vi "LOER_GetImage.vi"(0 "XRef":T5, 1 "State In":T3={"Inputs"=1, "SelectedIndex"=1, "ClassInfo"=[], "Width"=100, "EventReg Type"=variant}) -> (14 "Image":T2, 15 "Fatal Error Out":T1)   [LabVIEW 2016, in "LV Object Event Registration Node.xnode"]
uses:
  LV Object Event Registration Node.xnode
  <vilib>/XNodeSupport/XNodeXNodeRef.ctl
  LOER_State.ctl
  LOER_ClassInfo.ctl
  <vilib>/XNodeSupport/XNodeImage.ctl
  <vilib>/XNodeSupport/XNodeErrorCluster.ctl
  <vilib>/XNodeSupport/NI_XNodeSupport.lvlib
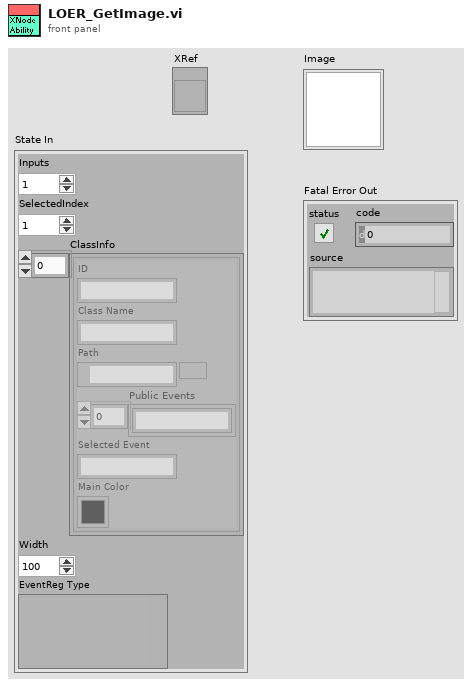
[diagram p1: front panel]
types:
  T1 = typedef "NI_XNodeSupport.lvlib/XNodeErrorCluster.ctl" = errorcluster
  T2 = typedef "NI_XNodeSupport.lvlib/XNodeImage.ctl" = picture
  T3 = typedef "LV Object Event Registration Node.xnode/LOER_State.ctl" = cluster{"Inputs":u16, "SelectedIndex":i16, "ClassInfo":T4[], "Width":u16, "EventReg Type":variant}
  T4 = typedef "LV Object Event Registration Node.xnode/LOER_ClassInfo.ctl" = cluster{"ID":string, "Class Name":string, "Path":path, "Public Events":string[], "Selected Event":string, "Main Color":u32}
  T5 = typedef "NI_XNodeSupport.lvlib/XNodeXNodeRef.ctl" = refnum<vi>
  T6 = cluster{"horizontal":enum16{"left", "center", "right"}, "vertical":enum16{"top", "center", "bottom"}}
  T7 = cluster{"left":i16, "top":i16, "right":i16, "bottom":i16}
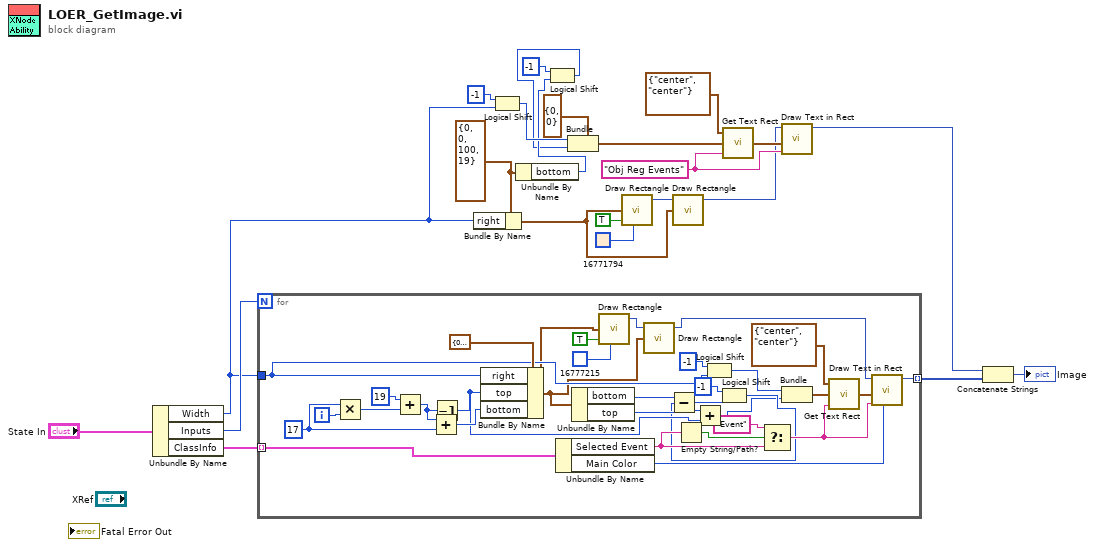
[diagram p0: block diagram]
diagram:
  w12 = "Obj Reg Events" ("text")
  w4 = T7 {"left"=0, "top"=0, "right"=100, "bottom"=19} ("rect")
  n1 = Unbundle By Name("State In") -> ("Width"=w8:u16, "Inputs"=w22:u16, "ClassInfo"=w17:T4[])
  n2 = for {
    N: w22 -> [_]
    tunnel: [w51] -> w18 mode=indexing
    tunnel: w17 -> [w41] mode=indexing
    tunnel: w8 -> [w33]
    i -> [w50]
    w45 = 17 ("x")
    n3 = Multiply(x=w45, y=w50) -> (x*y=w49:i32)
    n4 = Add(x=19, y=w49) -> (x+y=w46:i32)
    n5 = Add(x=w46, y=w45) -> (x+y=w44:i32)
    n6 = Decrement(x=w46) -> (x-1=w27:i32)
    n7 = Bundle By Name(cluster=T7 {"left"=0, "top"=0, "right"=100, "bottom"=0} ("rect"), "right"=w33, "top"=w27, "bottom"=w44) -> (w31:T7)
    n8 = Unbundle By Name(w41) -> ("Selected Event"=w39:string, "Main Color"=w36:u32)
    n9 = Unbundle By Name(w31) -> ("bottom"=w30:i16, "top"=w29:i16)
    n10 = call <vilib>:"Draw Rectangle.vi"("rect"=w31, "fill?(F)"=TRUE, "color(black)"=u32 16777215) -> ("new picture"=w35:picture)  [unwired: 6 in]
    n11 = call <vilib>:"Draw Rectangle.vi"("picture"=w35, "rect"=w31) -> ("new picture"=w34:picture)  [unwired: 7 in]
    n12 = Subtract(x=w30, y=w29) -> (x-y=w26:i16)
    n13 = Empty String/Path?(string/path=w39) -> (empty?=w40:bool)
    n14 = Logical Shift(y=i16 -1, x=w33) -> (x << y=w42:u16)
    n15 = Logical Shift(y=i16 -1, x=w26) -> (x << y=w25:i16)
    n16 = Add(x=w25, y=w27) -> (x+y=w24:i32)
    n17 = Select(t="Event" ("format string"), s=w40, f=w39) -> (s? t:f=w37:string)
    n18 = Bundle(w42, w24) -> (w32:cluster{u16, i32})  [unwired: 1 in]
    n19 = call <vilib>:"Get Text Rect.vi"("alignment(left, top)"=T6 {"horizontal"=enum."center", "vertical"=enum."center"}, "origin(0,0)"=w32, "text"=w37) -> ("rect"=w54:T7)  [unwired: 6 in]
    n20 = call <vilib>:"Draw Text in Rect.vi"("text color(black)"=w36, "text"=w37, "rect"=w54, "picture"=w34) -> ("new picture"=w51:picture)  [unwired: 7 in]
  }
  n21 = Bundle By Name(cluster=w4, "right"=w8) -> (w15:T7)
  n22 = Logical Shift(y=i16 -1, x=w8) -> (x << y=w6:u16)
  n23 = Unbundle By Name(w4) -> ("bottom"=w2:i16)
  n24 = Logical Shift(y=i16 -1, x=w2) -> (x << y=w1:i16)
  n25 = Bundle(cluster=cluster{"horizontal":i16, "vertical":i16} {"horizontal"=0, "vertical"=0} ("origin(0,0)"), "horizontal"=w6, "vertical"=w1) -> (w5:cluster{"horizontal":i16, "vertical":i16})
  n26 = call <vilib>:"Draw Rectangle.vi"("rect"=w15, "fill?(F)"=TRUE, "color(black)"=u32 16771794) -> ("new picture"=w16:picture)  [unwired: 6 in]
  n27 = call <vilib>:"Draw Rectangle.vi"("picture"=w16, "rect"=w15) -> ("new picture"=w11:picture)  [unwired: 7 in]
  n28 = call <vilib>:"Get Text Rect.vi"("alignment(left, top)"=T6 {"horizontal"=enum."center", "vertical"=enum."center"}, "origin(0,0)"=w5, "text"=w12) -> ("rect"=w14:T7)  [unwired: 6 in]
  n29 = call <vilib>:"Draw Text in Rect.vi"("text"=w12, "rect"=w14, "picture"=w11) -> ("new picture"=w10:picture)  [unwired: 8 in]
  n30 = Concatenate Strings(w10, w18) -> (→"Image":picture)
